vi "Launch Core.vi"(8 "error in (no error)":errorcluster, 9 "Negative Fit":refnum<class "Sinusoidal Fit.lvclass">, 10 "Positive Fit":refnum<class "Sinusoidal Fit.lvclass">, 11 "Halfwave Fit Display in":refnum<class "Halfwave Fit Display.lvclass">) -> (0 "error out":errorcluster, 3 "Halfwave Fit Display out":refnum<class "Halfwave Fit Display.lvclass">)   [LabVIEW 2016, in "Halfwave Fit Display.lvclass"]
uses:
  Halfwave Fit Display.lvclass
  Sinusoidal Fit/Sinusoidal Fit.lvclass
  Halfwave Fit Display.lvclass/Halfwave Fit Display.ctl
  Core.vi
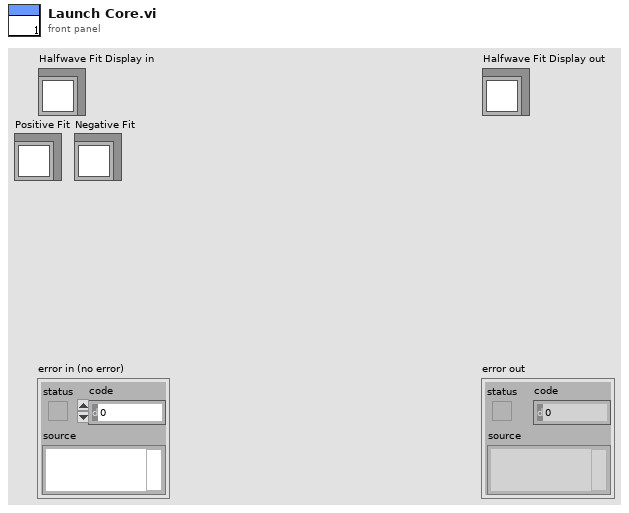
[diagram p1: front panel]
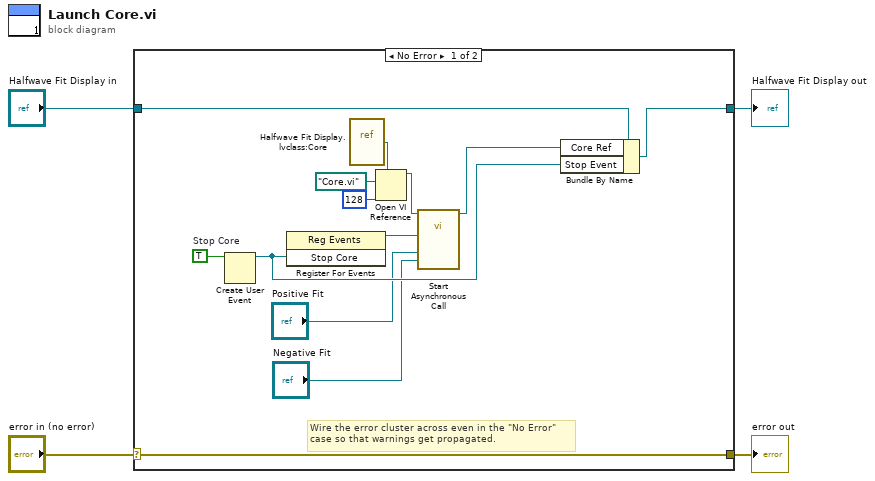
[diagram p0: block diagram]
diagram:
  n1 = case shown="No Error" "error in (no error)" {
    selector: "error in (no error)" -> [w17 w19]
    tunnel: [w17 w19] -> w3
    tunnel: [w12 w18] -> w1
    tunnel: "Halfwave Fit Display in" -> [w13 w18]
    frame No Error {
      w10 = TRUE  # Stop Core
      # "Wire the error cluster across even in the \"No Error\"\ncase so that warnings get propagated."
      n2 = Create User Event(user event datatype=w10) -> (user event=w7:refnum<user-event>)  [unwired: 1 in, 1 out]
      n3 = register-events(w7) -> (reference out=w9:refnum<event-registration>)  [unwired: 2 in, 1 out]
      n4 = vi-ref "Halfwave Fit Display.lvclass:Core.vi"() -> (w16:refnum<vi>)
      n5 = Open VI Reference(type specifier VI Refnum (for type only)=w16, vi path=path "Core.vi", options=128) -> (vi reference=w15:refnum<vi>)  [unwired: 3 in, 1 out]
      n6 = call-by-ref "Start Asynchronous Call"(reference=w15, "Negative Fit"="Negative Fit", "Positive Fit"="Positive Fit", "event registration refnum"=w9) -> (reference out=w8:refnum<vi>)  [unwired: 10 in, 1 out]
      n7 = Bundle By Name(cluster=w13, "Core Ref"=w8, "Stop Event"=w7) -> (w12:refnum<class "Halfwave Fit Display.lvclass">)
    }
    frame Error {
    }
  }
  "error out" <- w3
  "Halfwave Fit Display out" <- w1
